vi "Get Hilbert Compensation.vi"(11 "frequency":dbl) -> (3 "compensation value":dbl)   [LabVIEW 2017, in "Lock-In Amplifier Example Host.lvlib"]
uses:
  Lock-In Amplifier Example Host.lvlib
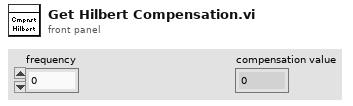
[diagram p1: front panel]
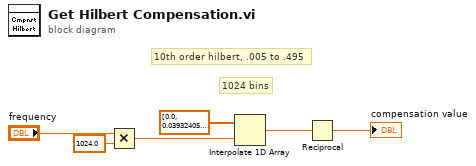
[diagram p0: block diagram]
diagram:
  # "1024 bins"
  # "10th order hilbert, .005 to .495"
  n1 = Multiply(x="frequency", y=1024.0) -> (x*y=w4:dbl)
  n2 = Interpolate 1D Array(1:w4, 2:dbl[] [0.0, 0.0393240571880461, 0.07862305577132073, 0.11787195881338744, 0.15704577269465517, 0.19611956872125783, 0.23506850467453408, 0.27386784628139277, 0.31249298858592484, 0.3509194772027122, 0.3891230294323973, 0.42707955522020186, 0.4647651779382325, 0.5021562549725738, 0.5392293980963521, 0.5759614936101493, 0.6123297222313703, 0.6483115787143895, 0.683884891183569, 0.7190278401614885, 0.7537189772750307, 0.787937243622251, 0.8216619877832846, 0.8548729834588719, 0.8875504467204313, 0.9196750528559701, 0.9512279527964993, 0.9821907891080112, 1.0125457115344798, 1.0422753920777643, 1.0713630396007292, 1.0997924139403306, 1.1275478395178837, 1.1546142184341897, 1.1809770430376783, 1.2066224079542163, 1.2315370215677324, 1.2557082169413156, 1.2791239621689732, 1.301772870148753, 1.3236442077684871, 1.3447279044959424, 1.3650145603657369, 1.3844954533559255, 1.403162546147736, 1.421008492262504, 1.4380266415704421, 1.4542110451664503, 1.469556459608778, 1.4840583505169216, 1.4977128955257601, 1.5105169865935049, 1.52246823166166, 1.533564955665777, 1.5438062008963993, 1.5531917267101956, 1.5617220085918713, 1.5693982365680708, 1.5762223129750663, 1.5821968495826355, 1.5873251640771324, 1.5916112759073393, 1.5950599014972835, 1.5976764488307988, 1.5994670114131706, 1.6004383616158047, 1.6005979434104198, 1.5999538644998237, 1.5985148878529045, 1.5962904226520118, 1.5932905146614411, 1.5895258360262814, 1.5850076745114088, 1.5797479221909114, 1.5737590635987697, 1.5670541633520736, 1.5596468532585797, 1.5515513189208692, 1.5427822858498257, 1.5333550051006262, 1.5232852384448479, 1.51258924309275, 1.5012837559801795, 1.4893859776349587, 1.4769135556380009, 1.463884567694768, 1.4503175043330367, 1.4362312512432902, 1.4216450712783673, 1.4065785861293238, 1.3910517576947452, 1.3750848691610298, 1.3586985058114298, 1.3419135355818739, 1.3247510893818286, 1.3072325411986654, 1.289379488004192, 1.2712137294821853, 1.2527572475959188, 1.2340321860148227, 1.2150608294195273, 1.1958655827046596, 1.1764689500988337, 1.156893514221353, 1.1371619150951926, 1.1172968291358532, 1.097320948135701, 1.0772569582633922, 1.0571275190979668, 1.0369552427171473, 1.0167626728593187, 0.9965722641785881, 0.9764063616122284, 0.9562871798796858, 0.9362367831322123, 0.9162770647720141, 0.8964297274596621, 0.876716263328301, 0.8571579344230053, 0.8377757533834062, 0.81859046438747, 0.7996225243740624, 0.7808920845616583, 0.7624189722802671, 0.7442226731333463, 0.7263223135061521, 0.7087366434366431, 0.6914840198647084, 0.6745823902751188, 0.6580492767492289, 0.6419017604400643, 0.6261564664850184, 0.6108295493699678, 0.5959366787581837, 0.5814930257969683, 0.5675132499144924, 0.5540114861188405, 0.5410013328107923, 0.528495840121375, 0.516507498784727, 0.5050482295562985, 0.4941293731858972, 0.48376168095455924, 0.47395530578368883, 0.46471979392436663, 0.45606407723417386, 0.4479964660483225, 0.44052464265131724, 0.43365565535480416, 0.42739591318668624, 0.4217511811960057, 0.41672657637751104, 0.4123265642192345, 0.40855495587582213, 0.40541490596975865, 0.40290891102204074, 0.401038808513252, 0.39980577657539995, 0.39921033431427383, 0.39925234276149163, 0.39993100645480456, 0.40124487564463246, 0.4031918491242209, 0.4057691776802061, 0.4089734681598043, 0.41280068815024784, 0.4172461712655174, 0.4223046230348482, 0.4279701273869147, 0.43423615372304425, 0.4410955645722468, 0.4485406238203061, 0.4565630055046323, 0.4651538031660465, 0.47430353974814066, 0.484002178034343, 0.4942391316123111, 0.5050032763547818, 0.5162829624055196, 0.528066026658528, 0.5403398057182334, 0.5530911493278886, 0.5663064342530129, 0.5799715786062526, 0.5940720565996385, 0.6085929137098062, 0.623518782241372, 0.6388338972732749, 0.6545221129725365, 0.6705669192595575, 0.6869514588087303, 0.7036585443678398, 0.7206706763794295, 0.7379700608870223, 0.7555386277088302, 0.7733580488613302, 0.7914097572148586, 0.8096749653631574, 0.8281346846886132, 0.846769744604746, 0.8655608119573434, 0.8844884105654953, 0.903532940883651, 0.9226746997657143, 0.9418939003121072, 0.9611706917806482, 0.9804851795420476, 0.9998174450607822, 1.019147565882089, 1.0384556356058272, 1.0577217838279678, 1.0769261960305117, 1.09604913340069, 1.1150709525603753, 1.133972125186722, 1.152733257505162, 1.1713351096360174, 1.1897586147761223, 1.2079848981970225, 1.2259952960414926, 1.2437713739003136, 1.261294945151464, 1.2785480890441108, 1.295513168510037, 1.3121728476853975, 1.3285101091259954, 1.3445082706995413, 1.360151002138696, 1.3754223412390059, 1.3903067096861927, 1.404788928497616, 1.418854233063096, 1.4324882877706695, 1.4456772002032583, 1.4584075348926326, 1.4706663266174855, 1.4824410932328698, 1.4937198480186944, 1.5044911115354556, 1.514743922975824, 1.5244678510012262, 1.5336530040530192, 1.542290040128393, 1.5503701760116213, 1.5578851959518265, 1.5648274597789367, 1.5711899104500666, 1.5769660810190875, 1.5821501010227137, 1.5867367022769887, 1.590721224078616, 1.5940996178061535, 1.596868450916668, 1.5990249103340182, 1.6005668052255204, 1.601492569164344, 1.6018012616755561, 1.601492569164344, 1.6005668052255204, 1.5990249103340182, 1.596868450916668, 1.5940996178061535, 1.590721224078616, 1.5867367022769887, 1.5821501010227137, 1.5769660810190875, 1.5711899104500666, 1.5648274597789367, 1.5578851959518265, 1.5503701760116217, 1.5422900401283932, 1.5336530040530199, 1.5244678510012266, 1.5147439229758246, 1.504491111535456, 1.493719848018695, 1.4824410932328702, 1.4706663266174862, 1.458407534892633, 1.4456772002032587, 1.43248828777067, 1.4188542330630964, 1.4047889284976165, 1.3903067096861932, 1.3754223412390063, 1.3601510021386967, 1.3445082706995417, 1.328510109125996, 1.312172847685398, 1.2955131685100374, 1.2785480890441114, 1.2612949451514643, 1.243771373900314, 1.225995296041493, 1.2079848981970231, 1.189758614776123, 1.1713351096360178, 1.1527332575051625, 1.1339721251867225, 1.1150709525603761, 1.096049133400691, 1.0769261960305125, 1.0577217838279687, 1.038455635605828, 1.0191475658820899, 0.9998174450607829, 0.9804851795420483, 0.9611706917806488, 0.9418939003121078, 0.9226746997657149, 0.9035329408836517, 0.8844884105654962, 0.8655608119573442, 0.8467697446047469, 0.8281346846886141, 0.8096749653631583, 0.7914097572148594, 0.773358048861331, 0.7555386277088308, 0.737970060887023, 0.7206706763794303, 0.7036585443678406, 0.686951458808731, 0.6705669192595582, 0.6545221129725373, 0.6388338972732757, 0.6235187822413728, 0.608592913709807, 0.5940720565996394, 0.5799715786062535, 0.5663064342530136, 0.5530911493278894, 0.5403398057182341, 0.5280660266585288, 0.5162829624055204, 0.5050032763547826, 0.49423913161231176, 0.4840021780343437, 0.47430353974814143, 0.4651538031660473, 0.4565630055046331, 0.44854062382030685, 0.4410955645722476, 0.43423615372304497, 0.4279701273869154, 0.42230462303484895, 0.4172461712655181, 0.41280068815024856, 0.40897346815980495, 0.40576917768020676, 0.4031918491242216, 0.4012448756446331, 0.3999310064548051, 0.3992523427614922, 0.3992103343142744, 0.3998057765754005, 0.4010388085132526, 0.4029089110220413, 0.4054149059697592, 0.4085549558758227, 0.4123265642192351, 0.4167265763775115, 0.4217511811960062, 0.4273959131866867, 0.4336556553548046, 0.44052464265131774, 0.44799646604832294, 0.4560640772341742, 0.4647197939243669, 0.47395530578368916, 0.4837616809545596, 0.4941293731858976, 0.5050482295562988, 0.5165074987847273, 0.5284958401213752, 0.5410013328107925, 0.5540114861188408, 0.5675132499144926, 0.5814930257969685, 0.5959366787581839, 0.6108295493699679, 0.6261564664850185, 0.6419017604400645, 0.658049276749229, 0.6745823902751189, 0.6914840198647085, 0.7087366434366431, 0.7263223135061521, 0.7442226731333463, 0.7624189722802671, 0.7808920845616583, 0.7996225243740624, 0.81859046438747, 0.8377757533834062, 0.8571579344230053, 0.876716263328301, 0.8964297274596621, 0.9162770647720139, 0.936236783132212, 0.9562871798796856, 0.9764063616122277, 0.9965722641785879, 1.0167626728593184, 1.036955242717147, 1.0571275190979663, 1.0772569582633917, 1.0973209481357005, 1.1172968291358527, 1.1371619150951922, 1.1568935142213526, 1.1764689500988332, 1.1958655827046591, 1.2150608294195269, 1.2340321860148222, 1.2527572475959183, 1.2712137294821848, 1.2893794880041916, 1.307232541198665, 1.3247510893818282, 1.3419135355818734, 1.3586985058114294, 1.3750848691610293, 1.3910517576947448, 1.4065785861293234, 1.4216450712783668, 1.4362312512432895, 1.4503175043330363, 1.4638845676947676, 1.4769135556380004, 1.4893859776349583, 1.5012837559801788, 1.5125892430927492, 1.5232852384448468, 1.5333550051006255, 1.542782285849825, 1.5515513189208685, 1.559646853258579, 1.567054163352073, 1.5737590635987693, 1.5797479221909108, 1.5850076745114081, 1.589525836026281, 1.5932905146614404, 1.5962904226520112, 1.5985148878529039, 1.5999538644998232, 1.6005979434104192, 1.6004383616158042, 1.5994670114131702, 1.5976764488307984, 1.595059901497283, 1.5916112759073386, 1.587325164077132, 1.582196849582635, 1.5762223129750659, 1.5693982365680703, 1.5617220085918708, 1.5531917267101951, 1.5438062008963989, 1.5335649556657767, 1.5224682316616596, 1.5105169865935044, 1.4977128955257597, 1.4840583505169211, 1.4695564596087771, 1.4542110451664498, 1.4380266415704417, 1.4210084922625035, 1.4031625461477355, 1.384495453355925, 1.3650145603657364, 1.344727904495942, 1.3236442077684865, 1.3017728701487525, 1.2791239621689727, 1.2557082169413152, 1.231537021567732, 1.2066224079542158, 1.1809770430376778, 1.1546142184341892, 1.1275478395178833, 1.0997924139403301, 1.0713630396007288, 1.0422753920777639, 1.0125457115344794, 0.9821907891080108, 0.951227952796499, 0.9196750528559698, 0.8875504467204309, 0.8548729834588715, 0.8216619877832843, 0.7879372436222507, 0.7537189772750303, 0.7190278401614881, 0.6838848911835687, 0.6483115787143893, 0.6123297222313698, 0.575961493610149, 0.5392293980963518, 0.5021562549725735, 0.4647651779382323, 0.4270795552202016, 0.3891230294323972, 0.3509194772027121, 0.3124929885859247, 0.27386784628139266, 0.23506850467453397, 0.19611956872125777, 0.1570457726946551, 0.11787195881338738, 0.0786230557713207, 0.03932405718804609, 0.0] ("Waveform Graph")) -> (0:w2:dbl)
  n3 = Reciprocal(x=w2) -> (1/x=→"compensation value":dbl)
